vi "Kx_b Compute.vi"(8 "error in":errorcluster, 11 "Model Data":T1 {"Matricies"."K" format="%#_6e"; "Matricies"."Dout" format="%#_6e"; "Matricies"."Bout" format="%#_6e"; "Matricies"."Aout" format="%#_6e"; "Matricies"."Dint" format="%#_6e"; "Matricies"."Bint" format="%#_6e"; "Matricies"."Aint" format="%#_6e"; "Constants"."Z" format="%^#_6e"}) -> (0 "error out":errorcluster, 3 "Model Data out":T1 {"Matricies"."K" format="%#_6e"; "Matricies"."Dout" format="%#_6e"; "Matricies"."Bout" format="%#_6e"; "Matricies"."Aout" format="%#_6e"; "Matricies"."Dint" format="%#_6e"; "Matricies"."Bint" format="%#_6e"; "Matricies"."Aint" format="%#_6e"; "Constants"."Z" format="%^#_6e"})   [LabVIEW 2022 SP3]
uses:
  Model Data.ctl
  PZT type.ctl
  Piezo_Discs.ctl
  LEM_Params.ctl
  Layer Properties.ctl
  Matricies.ctl
  <vilib>/Utility/error.llb/DialogType.ctl
  <vilib>/Analysis/baseanly.llb/A x Vector.vi
  <vilib>/Analysis/Matrix/Numeric/Conversions/Array To Matrix - RA2.vi
  <vilib>/Analysis/baseanly.llb/Real Inverse Matrix.vi
  <vilib>/Analysis/Matrix/NI_Matrix.lvlib
  <vilib>/Analysis/NI_AALBase.lvlib
panel:
  out "c":dbl[](array[numeric]) format="%#_6e"
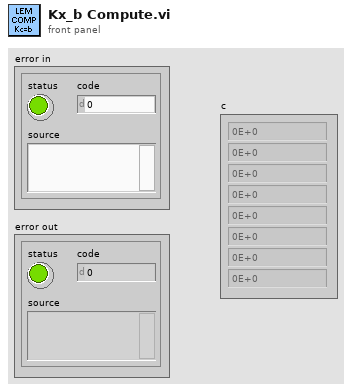
[diagram p1: front panel]
types:
  T1 = typedef "Model Data.ctl" = cluster{"Disc Properties":cluster{"Type":T2, "Disc Model":T3}, "Constants":cluster{"Radius":dbl[], "U(r)":dbl[], "W(r)":dbl[], "Vac":dbl, "P":dbl, "RiRo":dbl, "Area Density (r)":dbl[], "Ro":dbl, "Ri":dbl, "Z":dbl[], "Nr":dbl, "Mr":dbl, "c":dbl[], "AoC":dbl, "BoC":dbl, "AiC":dbl, "BiC":dbl, "f1":dbl, "f2":dbl}, "LEM Parameters":T4, "Layer Properties":T5[], "Matricies":T6}
  T2 = typedef "PZT type.ctl" = enum16{"Bimorph", "Unimorph"}
  T3 = typedef "Piezo_Discs.ctl" = enum16{"FTBD-21T-4.0A1", "PZT-5A (Gallas 1)", "PZT-5A (Gallas 2)", "AB4113B", "Create new disc...", "Load disc from file..."}
  T4 = typedef "LEM_Params.ctl" = cluster{"Displacement Ratio":dbl, "Cd":dbl, "Md":dbl, "xdc":dbl, "fd":dbl, "Sensitivity":dbl, "dA":dbl, "Rd":dbl, "Zeta":dbl, "Phi":dbl}
  T5 = typedef "Layer Properties.ctl" = cluster{"E":dbl, "R":dbl, "rho":dbl, "rhoA":dbl, "v":dbl, "A":dbl, "t":dbl, "d31":dbl, "size":enum16{"Outer", "Inner"}}
  T6 = typedef "Matricies.ctl" = cluster{"Aint":dbl[][], "Bint":dbl[][], "Dint":dbl[][], "Aout":dbl[][], "Bout":dbl[][], "Dout":dbl[][], "b":dbl[], "K":dbl[][]}
  T7 = typedef "DialogType.ctl" = u16
  T8 = typedef "NI_Matrix.lvlib/RealMatrix.ctl" = dbl[][]
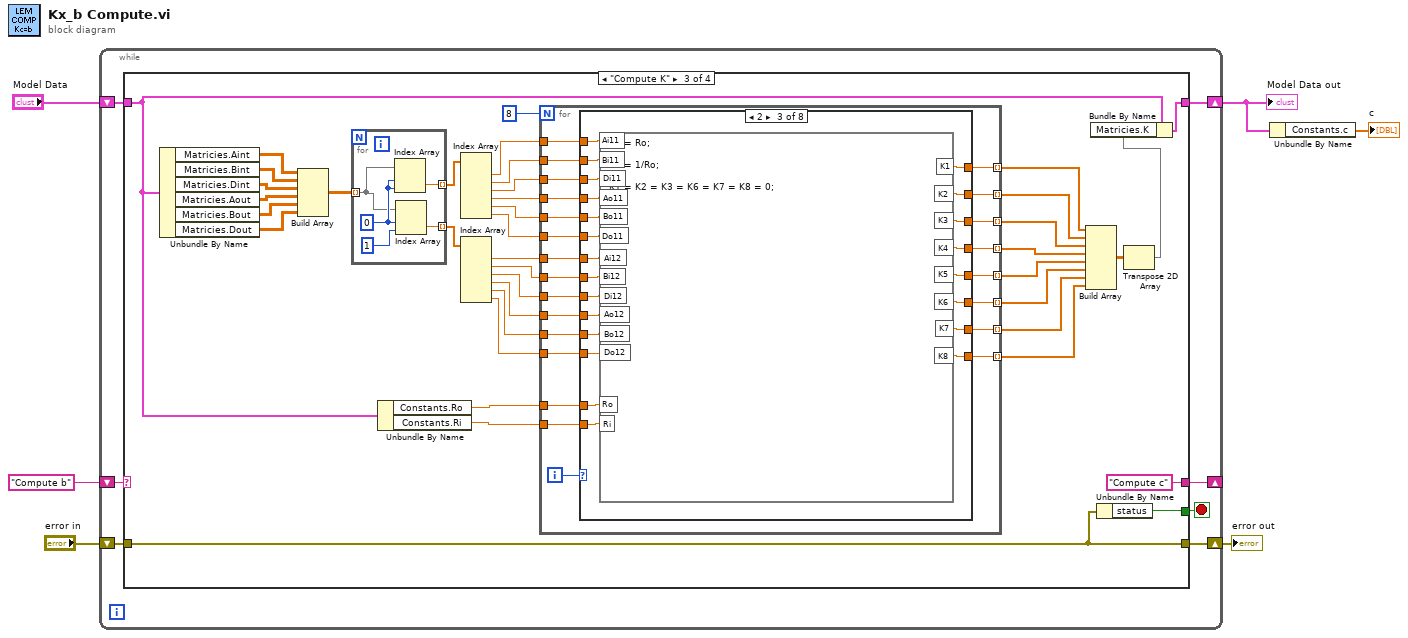
[diagram p0: block diagram]
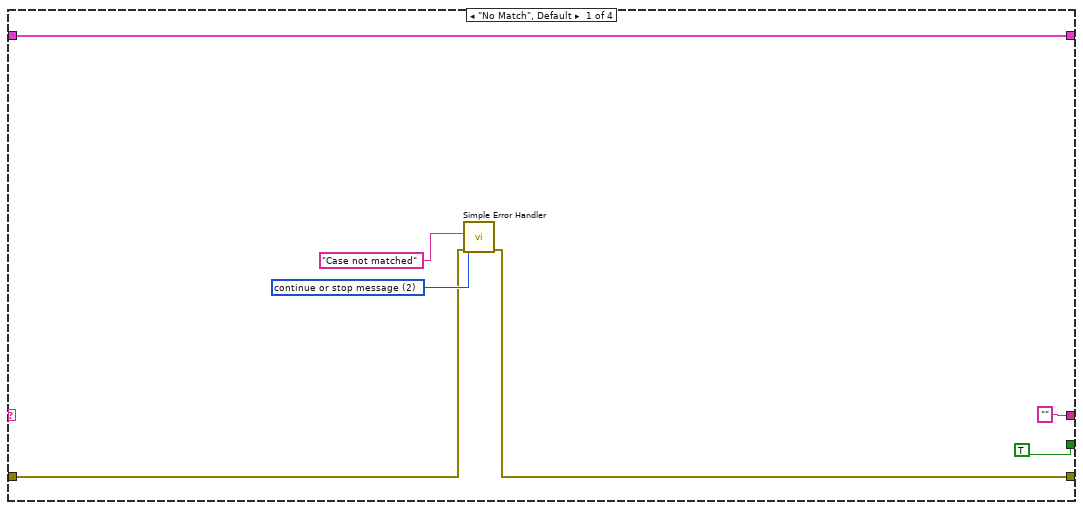
[diagram p2: hidden frame]
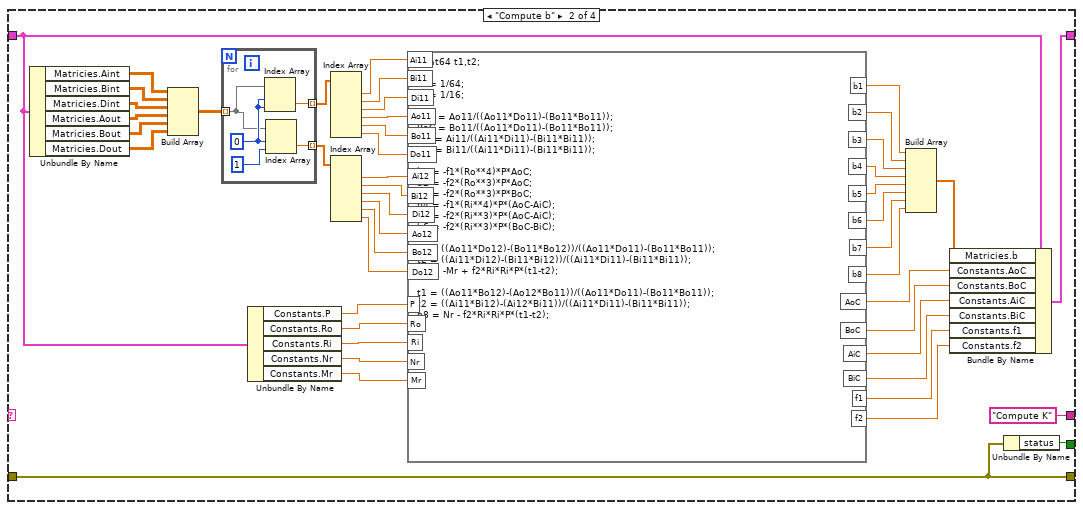
[diagram p3: hidden frame]
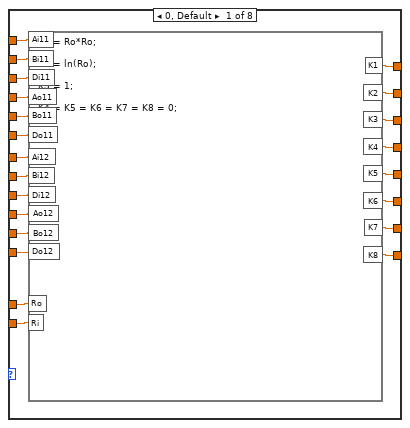
[diagram p4: hidden frame]
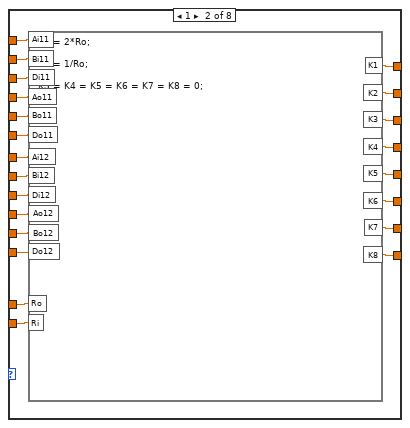
[diagram p5: hidden frame]
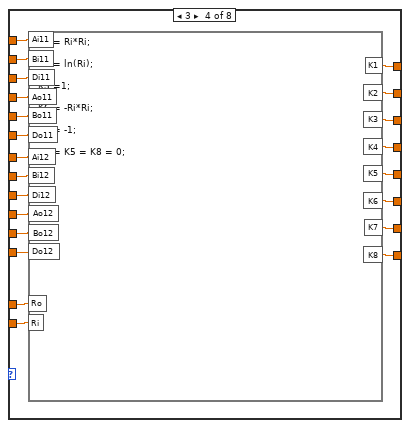
[diagram p6: hidden frame]
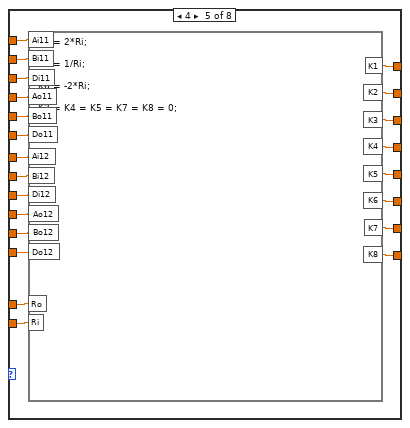
[diagram p7: hidden frame]
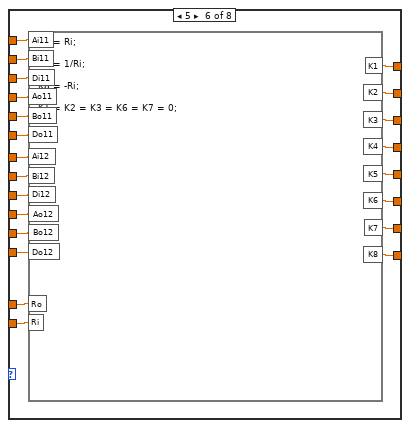
[diagram p8: hidden frame]
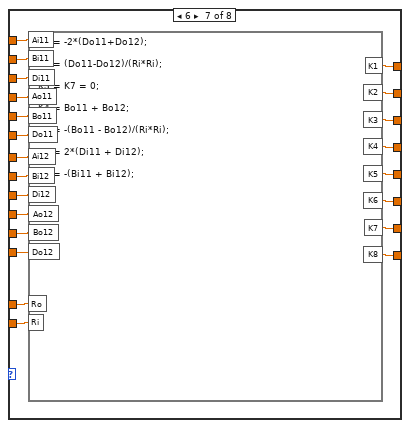
[diagram p9: hidden frame]
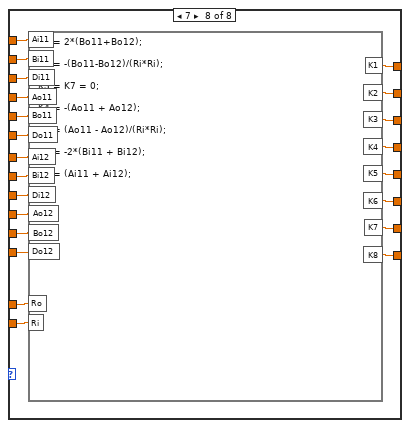
[diagram p10: hidden frame]
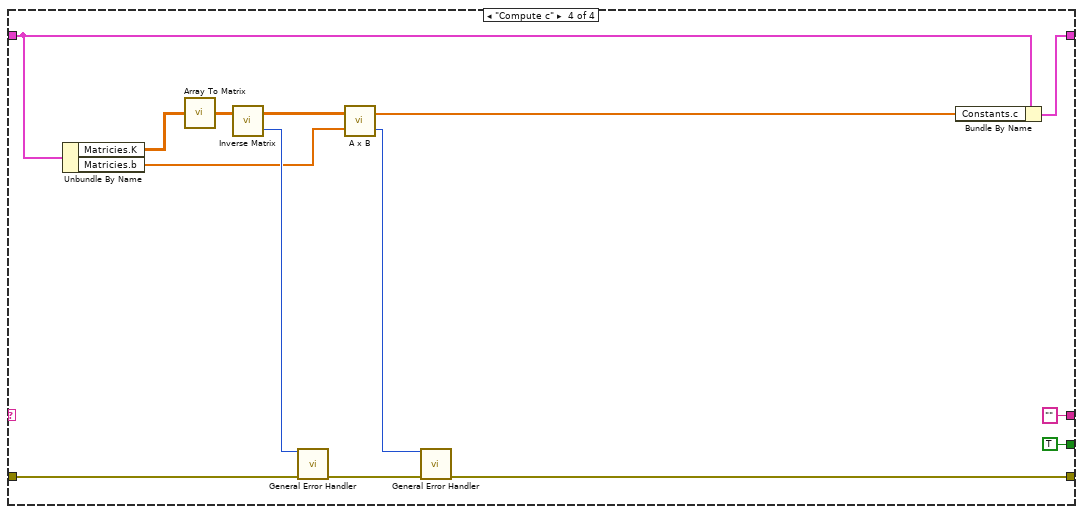
[diagram p11: hidden frame]
diagram:
  n1 = while {
    shift-right: [w10] -> _
    shift-left: "Compute b" -> [w11]
    shift-right: [w12] -> w2
    shift-left: "Model Data" -> [w9]
    shift-right: [w7] -> w4
    shift-left: "error in" -> [w8]
    stop <- w13 stop-if-true
    n2 = case shown="\"Compute K\"" w11 {
      tunnel: [TRUE w21 w72 TRUE] -> w13
      tunnel: [w16 w29 w84 w327] -> w12
      tunnel: ["" "Compute K" "Compute c" ""] -> w10
      tunnel: w9 -> [w16 w56 w85 w326]
      tunnel: w8 -> [w15 w22 w73 w318]
      tunnel: [w14 w22 w73 w325] -> w7
      frame "No Match", Default {
        w17 = T7 2 items=["no dialog", "OK message", "continue or stop message", "OK message + warnings", "continue/stop + warnings"] ("type of dialog (OK msg:1)")
        n3 = call <vilib>:"Simple Error Handler.vi"("error source (\" \")"="Case not matched", "type of dialog (OK msg:1)"=w17, "error in (no error)"=w15) -> ("error out"=w14:errorcluster)  [unwired: 2 in, 4 out]
      }
      frame "Compute b" {
        n4 = Unbundle By Name(w56) -> ("Matricies.Aint"=w65:dbl[][], "Matricies.Bint"=w64:dbl[][], "Matricies.Dint"=w63:dbl[][], "Matricies.Aout"=w62:dbl[][], "Matricies.Bout"=w61:dbl[][], "Matricies.Dout"=w60:dbl[][])
        n5 = Build Array(w65, w64, w63, w62, w61, w60) -> (w59:dbl[][][])
        n6 = for {
          tunnel: w59 -> [w69] mode=indexing
          tunnel: [w68] -> w58 mode=indexing
          tunnel: [w67] -> w57 mode=indexing
          w70 = 0 ("index (row)")
          n7 = Index Array(array=w69, index (row)=w70, index (col)=w70) -> (element=w68:dbl)
          n8 = Index Array(array=w69, index (row)=w70, index (col)=1) -> (element=w67:dbl)
        }
        n9 = Unbundle By Name(w56) -> ("Constants.P"=w34:dbl, "Constants.Ro"=w33:dbl, "Constants.Ri"=w32:dbl, "Constants.Nr"=w31:dbl, "Constants.Mr"=w30:dbl)
        n10 = Index Array(array=w58) -> (element #1=w46:dbl, element #2=w45:dbl, element #3=w44:dbl, element #4=w43:dbl, element #5=w42:dbl, element #6=w41:dbl)  [unwired: 6 in]
        n11 = Index Array(array=w57) -> (element #1=w40:dbl, element #2=w39:dbl, element #3=w38:dbl, element #4=w37:dbl, element #5=w36:dbl, element #6=w35:dbl)  [unwired: 6 in]
        n12 = formula code="float64 t1,t2;\n\nf1 = 1/64;\nf2 = 1/16;\n\nAoC = Ao11/((Ao11*Do11)-(Bo11*Bo11));\nBoC = Bo11/((Ao11*Do11)-(Bo11*Bo11));\nAiC = Ai11/((Ai11*Di11)-(Bi11*Bi11));\nBiC = Bi11/((Ai11*Di11)-(Bi11*Bi11));\n\nb1 = -f1*(Ro**4)*P*AoC;\nb2 = -f2*(Ro**3)*P*AoC;\nb3 = -f2*(Ro**3)*P*BoC;\nb4 = -f1*(Ri**4)*P*(AoC-AiC);\nb5 = -f2*(Ri**3)*P*(AoC-AiC);\nb6 = -f2*(Ri**3)*P*(BoC-BiC);\n\nt1 = ((Ao11*Do12)-(Bo11*Bo12))/((Ao11*Do11)-(Bo11*Bo11));\nt2 = ((Ai11*Di12)-(Bi11*Bi12))/((Ai11*Di11)-(Bi11*Bi11));\nb7 = -Mr + f2*Ri*Ri*P*(t1-t2);\n\nt1 = ((Ao11*Bo12)-(Ao12*Bo11))/((Ao11*Do11)-(Bo11*Bo11));\nt2 = ((Ai11*Bi12)-(Ai12*Bi11))/((Ai11*Di11)-(Bi11*Bi11));\nb8 = Nr - f2*Ri*Ri*P*(t1-t2);"("Ai11"=w46, "Bi11"=w45, "Di11"=w44, "Ao11"=w43, "Bo11"=w42, "Do11"=w41, "Ai12"=w40, "Bi12"=w39, "Di12"=w38, "Ao12"=w37, "Bo12"=w36, "Do12"=w35, "P"=w34, "Ro"=w33, "Ri"=w32, "Nr"=w31, "Mr"=w30) -> ("b1"=w54:dbl, "b2"=w53:dbl, "b3"=w52:dbl, "b4"=w51:dbl, "b5"=w50:dbl, "b6"=w49:dbl, "b7"=w48:dbl, "b8"=w47:dbl, "AoC"=w28:dbl, "BoC"=w27:dbl, "AiC"=w26:dbl, "BiC"=w25:dbl, "f1"=w24:dbl, "f2"=w23:dbl)
        n13 = Build Array(w54, w53, w52, w51, w50, w49, w48, w47) -> (w55:dbl[])
        n14 = Bundle By Name(cluster=w56, "Matricies.b"=w55, "Constants.AoC"=w28, "Constants.BoC"=w27, "Constants.AiC"=w26, "Constants.BiC"=w25, "Constants.f1"=w24, "Constants.f2"=w23) -> (w29:T1)
        n15 = Unbundle By Name(w22) -> ("status"=w21:bool)
      }
      frame "Compute K" {
        n16 = Unbundle By Name(w85) -> ("Matricies.Aint"=w109:dbl[][], "Matricies.Bint"=w108:dbl[][], "Matricies.Dint"=w107:dbl[][], "Matricies.Aout"=w106:dbl[][], "Matricies.Bout"=w105:dbl[][], "Matricies.Dout"=w104:dbl[][])
        n17 = Build Array(w109, w108, w107, w106, w105, w104) -> (w103:dbl[][][])
        n18 = for {
          tunnel: w103 -> [w312] mode=indexing
          tunnel: [w311] -> w102 mode=indexing
          tunnel: [w310] -> w101 mode=indexing
          w313 = 0 ("index (row)")
          n19 = Index Array(array=w312, index (row)=w313, index (col)=w313) -> (element=w311:dbl)
          n20 = Index Array(array=w312, index (row)=w313, index (col)=1) -> (element=w310:dbl)
        }
        n21 = Unbundle By Name(w85) -> ("Constants.Ro"=w88:dbl, "Constants.Ri"=w87:dbl)
        n22 = Index Array(array=w102) -> (element #1=w100:dbl, element #2=w99:dbl, element #3=w98:dbl, element #4=w97:dbl, element #5=w96:dbl, element #6=w95:dbl)  [unwired: 6 in]
        n23 = Index Array(array=w101) -> (element #1=w94:dbl, element #2=w93:dbl, element #3=w92:dbl, element #4=w91:dbl, element #5=w90:dbl, element #6=w89:dbl)  [unwired: 6 in]
        n24 = for {
          N: 8 -> [_]
          tunnel: w100 -> [w133]
          tunnel: w99 -> [w132]
          tunnel: w98 -> [w131]
          tunnel: w97 -> [w130]
          tunnel: w96 -> [w129]
          tunnel: w95 -> [w128]
          tunnel: w94 -> [w127]
          tunnel: w93 -> [w126]
          tunnel: w92 -> [w125]
          tunnel: w91 -> [w124]
          tunnel: w90 -> [w123]
          tunnel: w89 -> [w122]
          tunnel: w88 -> [w121]
          tunnel: w87 -> [w120]
          tunnel: [w119] -> w83 mode=indexing
          tunnel: [w118] -> w82 mode=indexing
          tunnel: [w117] -> w81 mode=indexing
          tunnel: [w116] -> w80 mode=indexing
          tunnel: [w115] -> w79 mode=indexing
          tunnel: [w114] -> w78 mode=indexing
          tunnel: [w113] -> w77 mode=indexing
          tunnel: [w112] -> w76 mode=indexing
          i -> [w111]
          n25 = case shown="2" w111 {
            tunnel: w133 -> [w155 w177 w199 w221 w243 w265 w287 w309]
            tunnel: w132 -> [w154 w176 w198 w220 w242 w264 w286 w308]
            tunnel: w131 -> [w153 w175 w197 w219 w241 w263 w285 w307]
            tunnel: w130 -> [w152 w174 w196 w218 w240 w262 w284 w306]
            tunnel: w129 -> [w151 w173 w195 w217 w239 w261 w283 w305]
            tunnel: w128 -> [w150 w172 w194 w216 w238 w260 w282 w304]
            tunnel: w127 -> [w149 w171 w193 w215 w237 w259 w281 w303]
            tunnel: w126 -> [w148 w170 w192 w214 w236 w258 w280 w302]
            tunnel: w125 -> [w147 w169 w191 w213 w235 w257 w279 w301]
            tunnel: w124 -> [w146 w168 w190 w212 w234 w256 w278 w300]
            tunnel: w123 -> [w145 w167 w189 w211 w233 w255 w277 w299]
            tunnel: w122 -> [w144 w166 w188 w210 w232 w254 w276 w298]
            tunnel: w121 -> [w143 w165 w187 w209 w231 w253 w275 w297]
            tunnel: w120 -> [w142 w164 w186 w208 w230 w252 w274 w296]
            tunnel: [w141 w163 w185 w207 w229 w251 w273 w295] -> w119
            tunnel: [w140 w162 w184 w206 w228 w250 w272 w294] -> w118
            tunnel: [w139 w161 w183 w205 w227 w249 w271 w293] -> w117
            tunnel: [w138 w160 w182 w204 w226 w248 w270 w292] -> w116
            tunnel: [w137 w159 w181 w203 w225 w247 w269 w291] -> w115
            tunnel: [w136 w158 w180 w202 w224 w246 w268 w290] -> w114
            tunnel: [w135 w157 w179 w201 w223 w245 w267 w289] -> w113
            tunnel: [w134 w156 w178 w200 w222 w244 w266 w288] -> w112
            frame 0, Default {
              n26 = formula code="K1 = Ro*Ro;\n\nK2 = ln(Ro);\n\nK3 = 1;\n\nK4 = K5 = K6 = K7 = K8 = 0;"("Ai11"=w155, "Bi11"=w154, "Di11"=w153, "Ao11"=w152, "Bo11"=w151, "Do11"=w150, "Ai12"=w149, "Bi12"=w148, "Di12"=w147, "Ao12"=w146, "Bo12"=w145, "Do12"=w144, "Ro"=w143, "Ri"=w142) -> ("K1"=w141:dbl, "K2"=w140:dbl, "K3"=w139:dbl, "K4"=w138:dbl, "K5"=w137:dbl, "K6"=w136:dbl, "K7"=w135:dbl, "K8"=w134:dbl)
            }
            frame 1 {
              n27 = formula code="K1 = 2*Ro;\n\nK2 = 1/Ro;\n\nK3 = K4 = K5 = K6 = K7 = K8 = 0;"("Ai11"=w177, "Bi11"=w176, "Di11"=w175, "Ao11"=w174, "Bo11"=w173, "Do11"=w172, "Ai12"=w171, "Bi12"=w170, "Di12"=w169, "Ao12"=w168, "Bo12"=w167, "Do12"=w166, "Ro"=w165, "Ri"=w164) -> ("K1"=w163:dbl, "K2"=w162:dbl, "K3"=w161:dbl, "K4"=w160:dbl, "K5"=w159:dbl, "K6"=w158:dbl, "K7"=w157:dbl, "K8"=w156:dbl)
            }
            frame 2 {
              n28 = formula code="K4 = Ro;\n\nK5 = 1/Ro;\n\nK1 = K2 = K3 = K6 = K7 = K8 = 0;"("Ai11"=w199, "Bi11"=w198, "Di11"=w197, "Ao11"=w196, "Bo11"=w195, "Do11"=w194, "Ai12"=w193, "Bi12"=w192, "Di12"=w191, "Ao12"=w190, "Bo12"=w189, "Do12"=w188, "Ro"=w187, "Ri"=w186) -> ("K1"=w185:dbl, "K2"=w184:dbl, "K3"=w183:dbl, "K4"=w182:dbl, "K5"=w181:dbl, "K6"=w180:dbl, "K7"=w179:dbl, "K8"=w178:dbl)
            }
            frame 3 {
              n29 = formula code="K1 = Ri*Ri;\n\nK2 = ln(Ri);\n\nK3 =1;\n\nK6 = -Ri*Ri;\n\nK7 = -1;\n\nK4 = K5 = K8 = 0;"("Ai11"=w221, "Bi11"=w220, "Di11"=w219, "Ao11"=w218, "Bo11"=w217, "Do11"=w216, "Ai12"=w215, "Bi12"=w214, "Di12"=w213, "Ao12"=w212, "Bo12"=w211, "Do12"=w210, "Ro"=w209, "Ri"=w208) -> ("K1"=w207:dbl, "K2"=w206:dbl, "K3"=w205:dbl, "K4"=w204:dbl, "K5"=w203:dbl, "K6"=w202:dbl, "K7"=w201:dbl, "K8"=w200:dbl)
            }
            frame 4 {
              n30 = formula code="K1 = 2*Ri;\n\nK2 = 1/Ri;\n\nK6 = -2*Ri;\n\nK3 = K4 = K5 = K7 = K8 = 0;"("Ai11"=w243, "Bi11"=w242, "Di11"=w241, "Ao11"=w240, "Bo11"=w239, "Do11"=w238, "Ai12"=w237, "Bi12"=w236, "Di12"=w235, "Ao12"=w234, "Bo12"=w233, "Do12"=w232, "Ro"=w231, "Ri"=w230) -> ("K1"=w229:dbl, "K2"=w228:dbl, "K3"=w227:dbl, "K4"=w226:dbl, "K5"=w225:dbl, "K6"=w224:dbl, "K7"=w223:dbl, "K8"=w222:dbl)
            }
            frame 5 {
              n31 = formula code="K4 = Ri;\n\nK5 = 1/Ri;\n\nK8 = -Ri;\n\nK1 = K2 = K3 = K6 = K7 = 0;"("Ai11"=w265, "Bi11"=w264, "Di11"=w263, "Ao11"=w262, "Bo11"=w261, "Do11"=w260, "Ai12"=w259, "Bi12"=w258, "Di12"=w257, "Ao12"=w256, "Bo12"=w255, "Do12"=w254, "Ro"=w253, "Ri"=w252) -> ("K1"=w251:dbl, "K2"=w250:dbl, "K3"=w249:dbl, "K4"=w248:dbl, "K5"=w247:dbl, "K6"=w246:dbl, "K7"=w245:dbl, "K8"=w244:dbl)
            }
            frame 6 {
              n32 = formula code="K1 = -2*(Do11+Do12);\n\nK2 = (Do11-Do12)/(Ri*Ri);\n\nK3 = K7 = 0;\n\nK4 = Bo11 + Bo12;\n\nK5 = -(Bo11 - Bo12)/(Ri*Ri);\n\nK6 = 2*(Di11 + Di12);\n\nK8 = -(Bi11 + Bi12);"("Ai11"=w287, "Bi11"=w286, "Di11"=w285, "Ao11"=w284, "Bo11"=w283, "Do11"=w282, "Ai12"=w281, "Bi12"=w280, "Di12"=w279, "Ao12"=w278, "Bo12"=w277, "Do12"=w276, "Ro"=w275, "Ri"=w274) -> ("K1"=w273:dbl, "K2"=w272:dbl, "K3"=w271:dbl, "K4"=w270:dbl, "K5"=w269:dbl, "K6"=w268:dbl, "K7"=w267:dbl, "K8"=w266:dbl)
            }
            frame 7 {
              n33 = formula code="K1 = 2*(Bo11+Bo12);\n\nK2 = -(Bo11-Bo12)/(Ri*Ri);\n\nK3 = K7 = 0;\n\nK4 = -(Ao11 + Ao12);\n\nK5 = (Ao11 - Ao12)/(Ri*Ri);\n\nK6 = -2*(Bi11 + Bi12);\n\nK8 = (Ai11 + Ai12);"("Ai11"=w309, "Bi11"=w308, "Di11"=w307, "Ao11"=w306, "Bo11"=w305, "Do11"=w304, "Ai12"=w303, "Bi12"=w302, "Di12"=w301, "Ao12"=w300, "Bo12"=w299, "Do12"=w298, "Ro"=w297, "Ri"=w296) -> ("K1"=w295:dbl, "K2"=w294:dbl, "K3"=w293:dbl, "K4"=w292:dbl, "K5"=w291:dbl, "K6"=w290:dbl, "K7"=w289:dbl, "K8"=w288:dbl)
            }
          }
        }
        n34 = Build Array(w83, w82, w81, w80, w79, w78, w77, w76) -> (w75:dbl[][])
        n35 = Unbundle By Name(w73) -> ("status"=w72:bool)
        n36 = Transpose 2D Array(2D array=w75) -> (transposed array=w74:dbl[][])
        n37 = Bundle By Name(cluster=w85, "Matricies.K"=w74) -> (w84:T1)
      }
      frame "Compute c" {
        n38 = Unbundle By Name(w326) -> ("Matricies.K"=w323:dbl[][], "Matricies.b"=w315:dbl[])
        n39 = call-poly <vilib>:"Array To Matrix.vi"("Real 2D Array"=w323) -> ("Real Matrix"=w322:T8)
        n40 = call-poly <vilib>:"Inverse Matrix.vi"("Input Matrix"=w322) -> ("error"=w316:i32, "Inverse Matrix"=w321:T8)  [unwired: 1 in]
        n41 = call <vilib>:"General Error Handler.vi"("[error code] (0)"=w316, "error in (no error)"=w318) -> ("error out"=w317:errorcluster)  [unwired: 9 in, 4 out]
        n42 = call-poly <vilib>:"A x B.vi"("Vector"=w315, "A"=w321) -> ("error"=w319:i32, "A x Vector"=w320:dbl[])
        n43 = call <vilib>:"General Error Handler.vi"("[error code] (0)"=w319, "error in (no error)"=w317) -> ("error out"=w325:errorcluster)  [unwired: 9 in, 4 out]
        n44 = Bundle By Name(cluster=w326, "Constants.c"=w320) -> (w327:T1)
      }
    }
  }
  "error out" <- w4
  "Model Data out" <- w2
  n45 = Unbundle By Name(w2) -> ("Constants.c"=→"c":dbl[])
